vi "Get LVClass Name from Data String.vi"(8 "error in":errorcluster, 10 "LVClass Data String":string) -> (0 "error out":errorcluster, 2 "LVClass Name":string)   [LabVIEW 2011, in "VITesterUtilities.lvlib"]
uses:
  Libraries/VITesterUtilities.lvlib
panel:
  # "Copyright © 2007 James Kring, Inc. All rights reserved.\n\nAuthor: Jim Kring <jim.kring@jameskring.com>\n\nThis library is provided \"AS IS\" , WITHOUT WARRANTIES OR \nCONDITIONS OF ANY KIND, either express or implied.\n\nJames Kring, Inc. -- http://www.jameskring.com"
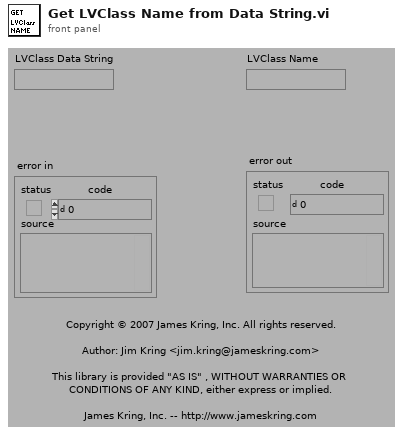
[diagram p1: front panel]
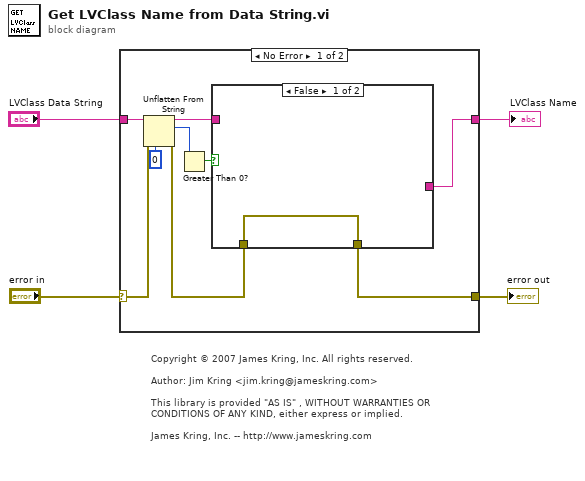
[diagram p0: block diagram]
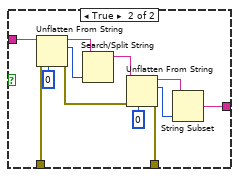
[diagram p2: hidden frame]
diagram:
  # "Copyright © 2007 James Kring, Inc. All rights reserved.\n\nAuthor: Jim Kring <jim.kring@jameskring.com>\n\nThis library is provided \"AS IS\" , WITHOUT WARRANTIES OR \nCONDITIONS OF ANY KIND, either express or implied.\n\nJames Kring, Inc. -- http://www.jameskring.com"
  n1 = case shown="No Error" "error in" {
    selector: "error in" -> [w7 w27]
    tunnel: [w11 _] -> w4
    tunnel: "LVClass Data String" -> [w10 _]
    tunnel: [w5 w27] -> w2
    frame No Error {
      n2 = Unflatten From String(type=u32 0, binary string=w10, error in (no error)=w7) -> (rest of the binary string=w9:string, value=w12:u32, error out=w6:errorcluster)  [unwired: 2 in]
      n3 = Greater Than 0?(x=w12) -> (x > 0?=w13:bool)
      n4 = case shown="False" w13 {
        tunnel: w9 -> [_ w26]
        tunnel: [_ w18] -> w11
        tunnel: [w14 w16] -> w5
        tunnel: w6 -> [w14 w15]
        frame False {
        }
        frame True {
          n5 = Unflatten From String(type=u8 0, binary string=w26, error in (no error)=w15) -> (rest of the binary string=w20:string, value=w21:u8, error out=w17:errorcluster)  [unwired: 2 in]
          n6 = Search/Split String(string=w20, offset (0)=w21) -> (substring before match=w19:string)  [unwired: 1 in, 2 out]
          n7 = Unflatten From String(type=u8 0, binary string=w19, error in (no error)=w17) -> (rest of the binary string=w23:string, value=w24:u8, error out=w16:errorcluster)  [unwired: 2 in]
          n8 = String Subset(string=w23, length (rest)=w24) -> (substring=w18:string)  [unwired: 1 in]
        }
      }
    }
    frame Error {
    }
  }
  "LVClass Name" <- w4
  "error out" <- w2
